vi "LiftEncoder.vi"() -> ()   [LabVIEW 2010]
uses:
  <vilib>/NXT/Subs/MotorXNode.DC Motor Type.ctl
  <vilib>/NXT/Subs/LVHSConnector.ctl
  <vilib>/NXT/NXTIO Xnodes/NXTIOXNode/NXTIO.xnode
  <vilib>/NXT/Subs/MotorXNode.1DCMotor.ctl
  <vilib>/NXT/NXTIO Xnodes/NXTIONodeSubVIs/TETRIX IO Reset Encoders.vi
  <vilib>/NXT/NXTIO Xnodes/AddressXNode/NXTIOAddress.xnode
  <vilib>/NXT/NXTIO Xnodes/NXTIONodeSubVIs/TETRIX IO Move a Fixed Distance.vi
  <vilib>/NXT/NXTIO Xnodes/NXTIONodeSubVIs/TETRIX IO Move DC Motors.vi
  <vilib>/NXT/NXTIO Xnodes/NXTIONodeSubVIs/TETRIX IO Motor Status.vi
panel:
  out "Curent Position":i32
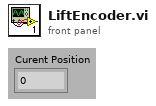
[diagram p1: front panel]
types:
  T1 = typedef "LVHSConnector.ctl" = cluster{"Hardware":string, "Flattened String":string}
  T2 = typedef "MotorXNode.DC Motor Type.ctl" = enum16{"DC Motor"}
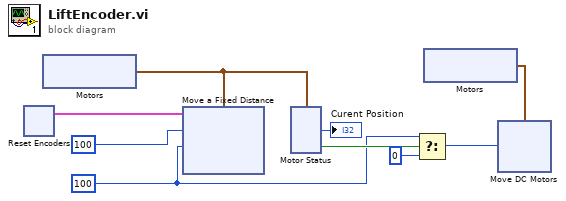
[diagram p0: block diagram]
diagram:
  w4 = 100 ("Power")
  n1 = xnode "Reset Encoders"() -> ("NXT"=w8:T1)  [unwired: 2 in]
  n2 = xnode "Motors"() -> ("DC Motor"=w1:cluster{"DC Motor":T2, "Address":i16})
  n3 = xnode "Move a Fixed Distance"("Speed 1"=w4, "Distance 1"=100 ("Go to Position"), "Motors"=w1, "NXT"=w8) -> ()  [unwired: 1 out]
  n4 = xnode "Motor Status"("Motors"=w1) -> ("Moving 1"=w5:bool, "Position 1"=→"Curent Position":i32)  [unwired: 1 in, 1 out]
  n5 = Select(t=w4, s=w5, f=0) -> (s? t:f=w2:i32)
  n6 = xnode "Motors"() -> ("DC Motor"=w6:cluster{"DC Motor":T2, "Address":i16})
  n7 = xnode "Move DC Motors"("Power/Speed 1"=w2, "Motors"=w6) -> ()  [unwired: 1 in, 1 out]
